vi "Vol-Viewer UI initialisation.vi"(5 "Source number of frames":T2(ring), 8 "error in (no error)":errorcluster) -> (0 "error out":errorcluster, 2 "Number of Frames":u32, 3 "Image ref":T1, 4 "Scrollbar position":i32)   [LabVIEW 2017]
uses:
  <vilib>/vision/Image Controls.llb/IMAQ Image.ctl
  Timelapse Viewer/Globals/gl_Time series viewer globals.vi
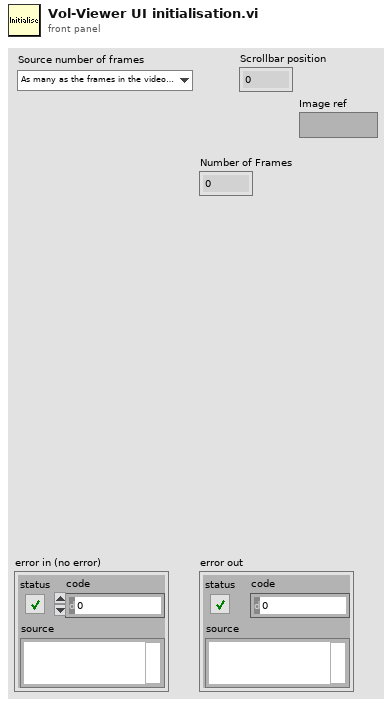
[diagram p1: front panel]
types:
  T1 = typedef "IMAQ Image.ctl" = refnum<image>
  T2 = enum16{"As many as the frames in the video with the fewest frames", "As many as the number of cycles"}
  T3 = enum8{"Enabled", "Disabled", "Disabled and Grayed Out"}
  T4 = typedef "Time series viewer refs.ctl" = cluster{"This VI":refnum<vi>, "Image control":refnum<vi>, "AVI Mode ind":refnum<vi>, "Play":refnum<vi>, "Stop":refnum<vi>, "Back":refnum<vi>, "Scrollbar":refnum<vi>, "Video length info":refnum<vi>, "Expected speed values":refnum<vi>, "Intensity":refnum<vi>, "Path":refnum<vi>, "Selection sliders":refnum<vi>, "Speed Graph ref":refnum<vi>, "Frame rate set (fps)":refnum<vi>, "Channel to load":refnum<vi>, "Number of rows to generate":refnum<vi>, "Colour":refnum<vi>}
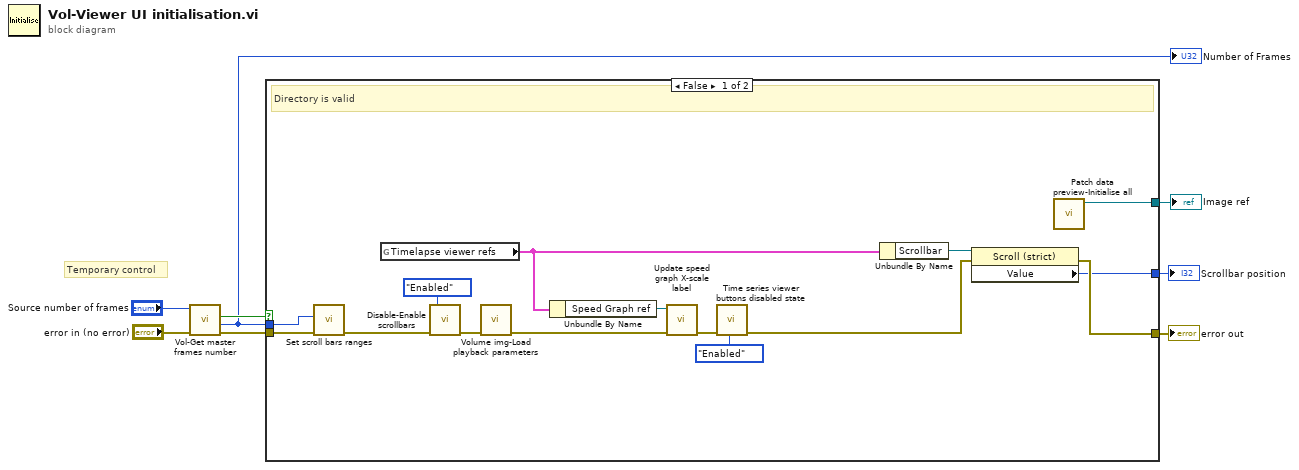
[diagram p0: block diagram]
diagram:
  # "Temporary control"
  n1 = call "Vol-Get master frames number.vi"("Source number of frames"="Source number of frames", "error in (no error)"="error in (no error)") -> ("error out"=w7:errorcluster, "Number of Frames"=w4:u32, "Cancelled due to the selected \nAVI file being located within an\n\"Exported 8-bit videos\" directory!"=w5:bool)  [unwired: 6 in, 1 out]
  "Number of Frames" <- w4
  n2 = case shown="False" w5 {
    tunnel: w7 -> [w23 w24]
    tunnel: w4 -> [w22 _]
    tunnel: [w21 w24] -> w6
    tunnel: [w20 _] -> w2
    tunnel: [w19 _] -> w1
    frame False {
      # "Directory is valid"
      n3 = call "Set scroll bars ranges.vi"("error in (no error)"=w23, "Number of frames"=w22) -> ("error out"=w9:errorcluster)  [unwired: 9 in]
      n4 = global read "gl_Time series viewer globals.vi" "Timelapse viewer refs"() -> (w14:T4)
      n5 = call "Disable-Enable scrollbars.vi"("error in (no error)"=w9, "Disabled state"=T3."Enabled") -> ("error out"=w17:errorcluster)  [unwired: 9 in]
      n6 = call "Volume img-Load playback parameters.vi"("error in (no error)"=w17) -> ("error out"=w13:errorcluster)  [unwired: 9 in, 1 out]
      n7 = Unbundle By Name(w14) -> ("Speed Graph ref"=w16:refnum<vi>)
      n8 = call "Update speed graph X-scale label.vi"("error in (no error)"=w13, "Speed Graph"=w16) -> ("error out"=w11:errorcluster)  [unwired: 9 in]
      n9 = call "Time series viewer buttons disabled state.vi"("error in (no error)"=w11, "Disabled"=T3."Enabled") -> ("error out"=w10:errorcluster)  [unwired: 9 in]
      n10 = Unbundle By Name(w14) -> ("Scrollbar"=w15:refnum<vi>)
      n11 = property class="Scroll (strict)"(reference=w15, error in=w10) -> (error out=w21:errorcluster, "Value"=w20:i32)  [unwired: 1 out]
      n12 = call "Patch data preview-Initialise all.vi"() -> ("U8 Image ref"=w19:T1)  [unwired: 11 in]
    }
    frame True {
      # "Cancelled due to the selected AVI file being located within an \"Exported 8-bit videos\" directory!"
    }
  }
  "error out" <- w6
  "Scrollbar position" <- w2
  "Image ref" <- w1
